vi "Teleop.vi"(10 "Match Info":T12={"Autonomous Elapsed Seconds"=0.0, "TeleOp Elapsed Seconds"=0.0, "Disabled Elapsed Seconds"=0.0, "Visited Autonomous"=FALSE, "Visited TeleOp"=FALSE, "Visited Disabled"=FALSE, "Autonomous Settings"={"Autonomous Style"=enum."Independent", "VI Refnum"=refnum}}, 11 "Call Context":T13) -> ()   [LabVIEW 2016]
doc: "This VI is called for each TeleOp packet received from the DS where the robot is not disabled. It is often used to read from the joysticks and update I/O or to update setpoints for timed control loops. It should complete and return within 20 milliseconds or it may miss DS packets."
uses:
  <vilib>/Rock Robotics/WPI/DriverStation/WPI_DriverStationDerivedRobotMode.ctl
  <vilib>/Rock Robotics/WPI/DriverStation/WPI_DriverStationMatch Info.ctl
  NavX/_TypeDefs/Flags/Z900_navX_Flags_OpStatusTypeDef.ctl
  NavX/_TypeDefs/Flags/Z900_navX_Flags_CalibrationStatusTypeDef.ctl
  NavX/_TypeDefs/Flags/Z900_navX_Flags_HardwareRevTypeDef.ctl
  NavX/_TypeDefs/Flags/Z900_navX_Flags_OmnimountConfigTypeDef.ctl
  NavX/_TypeDefs/FRIC_navX_DeviceNumbersTypeDef.ctl
  <vilib>/Rock Robotics/WPI/Utilities/WPI_GetSetVariantRefNum.vi
  <vilib>/Rock Robotics/Network Tables/NT Write Boolean Array.vi
  <vilib>/Rock Robotics/Network Tables/NT Write Numeric Array.vi
  <vilib>/Rock Robotics/Network Tables/NT Write Boolean.vi
  <vilib>/Rock Robotics/Network Tables/NT Read Boolean.vi
  <vilib>/Rock Robotics/Network Tables/NT Read Number.vi
  <vilib>/Rock Robotics/WPI/RobotDrive/WPI_RobotDriveMecanumDrive_Cartesian.vi
panel:
  out "YRPHfH 2":T1
  out "comp yaw 1":dbl format="%#.2f"
  out "Elapsed Time (s)":dbl
  out "comp yaw o":dbl format="%#.2f"
  in  "Zero Yaw":bool
  out "Displacement":T2 {"Velocity X" format="%.8f"; "Velocity Y" format="%.8f"; "Velocity Z" format="%.8f"; "Displace X" format="%.8f"; "Displace Y" format="%.8f"; "Displace Z" format="%.8f"}
  out "MPUTemp":dbl
  out "Board Information":T5 {"Board"."Hardware Revision" items=["navX-MXP"=33, "navX-Micro"=40]; "Omnimount Config" items=["DEFAULT", "X_UP", "X_DOWN", "Y_UP", "Y_DOWN", "Z_UP", "Z_DOWN"]}
  out "Linear Acceleration":cluster{"X":dbl, "Y":dbl, "Z":dbl} {"X" format="%_3g"; "Y" format="%_3g"; "Z" format="%_3g"}
  out "Offsets":T6 {"Yaw" format="%.8f"; "Quat W" format="%.8f"; "Quat X" format="%.8f"; "Quat Y" format="%.8f"; "Quat Z" format="%.8f"}
  out "Quaternion":T7 {"Quat W" format="%.8f"; "Quat X" format="%.8f"; "Quat Y" format="%.8f"; "Quat Z" format="%.8f"}
  out "Status":T10 {"OP Status" items=["INITIALIZING", "SELFTEST_IN_PROGRESS", "ERROR", "IMU_AUTOCAL_IN_PROGRESS", "NORMAL"]; "Calibration Status" items=["IMU_CAL_STATE_MASK"=3, "IMU_CAL_STATE_INPROGRESS"=0, "IMU_CAL_STATE_ACCUMULATE"=1, "IMU_CAL_STATE_COMPLETE"=2]}
  out "YRPHfH":T1
  out "Timestamp":u32
  out "Raw Values":T11 {"Accel X" format="%.8f"; "Accel Y" format="%.8f"; "Accel Z" format="%.8f"; "Gyro X" format="%.8f"; "Gyro Y" format="%.8f"; "Gyro Z" format="%.8f"; "Mag X" format="%.8f"; "Mag Y" format="%.8f"; "Mag Z" format="%.8f"}
  out "Sample Slider 0":dbl(slide) scale=0.0..5.0
  out "Sample Boolean 1":bool
  out "Sample Boolean 0":bool
  # "NavX"
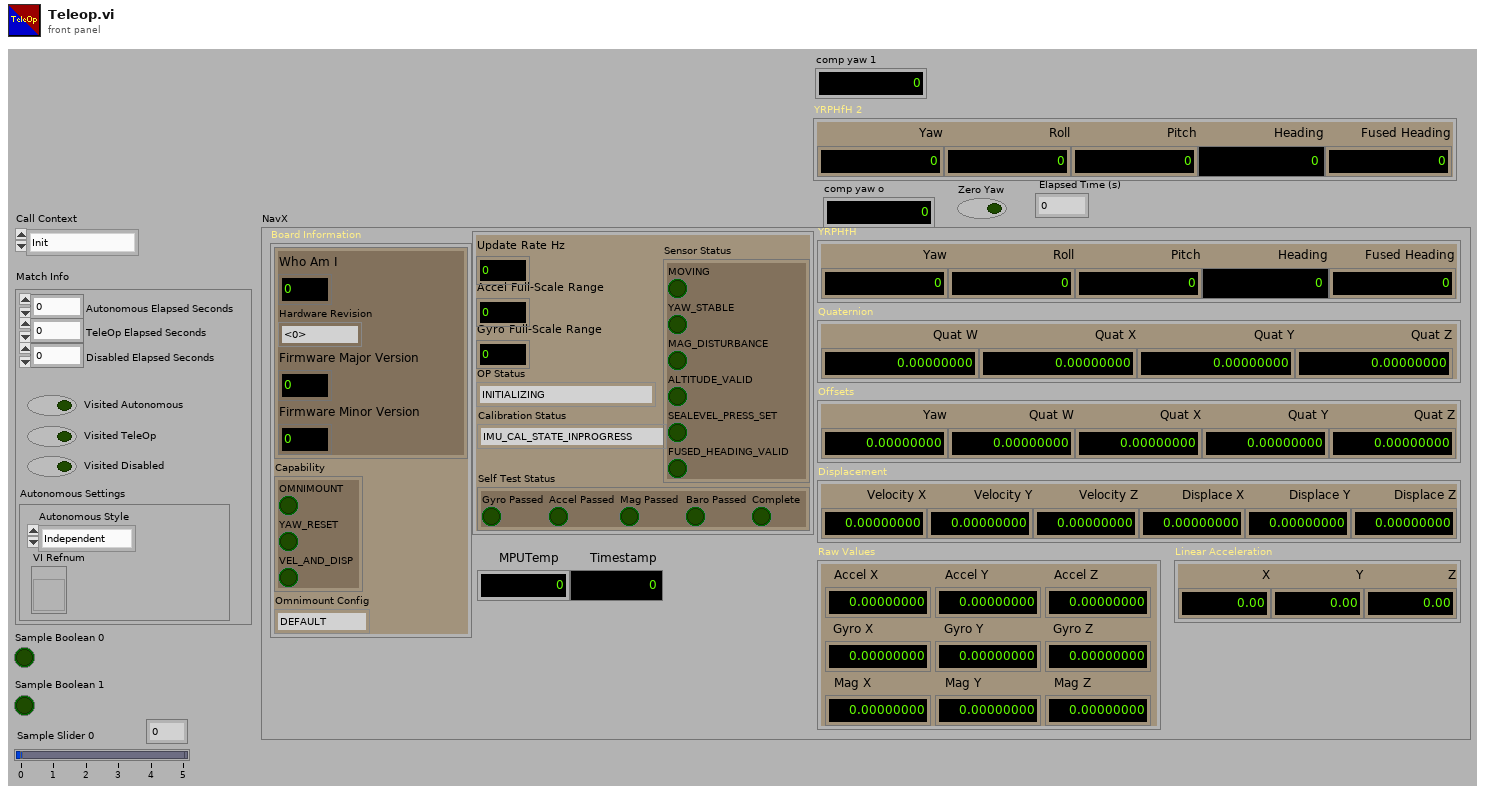
[diagram p1: front panel]
types:
  T1 = cluster{"Yaw":dbl, "Roll":dbl, "Pitch":dbl, "Heading":dbl, "Fused Heading":dbl}
  T2 = cluster{"Velocity X":dbl, "Velocity Y":dbl, "Velocity Z":dbl, "Displace X":dbl, "Displace Y":dbl, "Displace Z":dbl}
  T3 = typedef "Z900_navX_Flags_HardwareRevTypeDef.ctl" = u8
  T4 = typedef "Z900_navX_Flags_OmnimountConfigTypeDef.ctl" = u8
  T5 = cluster{"Board":cluster{"Who Am I":u8, "Hardware Revision":T3, "Firmware Major Version":u8, "Firmware Minor Version":u8}, "Capability":cluster{"OMNIMOUNT":bool, "YAW_RESET":bool, "VEL_AND_DISP":bool}, "Omnimount Config":T4}
  T6 = cluster{"Yaw":dbl, "Quat W":dbl, "Quat X":dbl, "Quat Y":dbl, "Quat Z":dbl}
  T7 = cluster{"Quat W":dbl, "Quat X":dbl, "Quat Y":dbl, "Quat Z":dbl}
  T8 = typedef "Z900_navX_Flags_OpStatusTypeDef.ctl" = u8
  T9 = typedef "Z900_navX_Flags_CalibrationStatusTypeDef.ctl" = u8
  T10 = cluster{"Update Rate Hz":u8, "Accel Full-Scale Range":u8, "Gyro Full-Scale Range":u16, "OP Status":T8, "Calibration Status":T9, "Sensor Status":cluster{"MOVING":bool, "YAW_STABLE":bool, "MAG_DISTURBANCE":bool, "ALTITUDE_VALID":bool, "SEALEVEL_PRESS_SET":bool, "FUSED_HEADING_VALID":bool}, "Self Test Status":cluster{"Gyro Passed":bool, "Accel Passed":bool, "Mag Passed":bool, "Baro Passed":bool, "Complete":bool}}
  T11 = cluster{"Accel X":dbl, "Accel Y":dbl, "Accel Z":dbl, "Gyro X":dbl, "Gyro Y":dbl, "Gyro Z":dbl, "Mag X":dbl, "Mag Y":dbl, "Mag Z":dbl}
  T12 = typedef "WPI_DriverStationMatch Info.ctl" = cluster{"Autonomous Elapsed Seconds":dbl, "TeleOp Elapsed Seconds":dbl, "Disabled Elapsed Seconds":dbl, "Visited Autonomous":bool, "Visited TeleOp":bool, "Visited Disabled":bool, "Autonomous Settings":cluster{"Autonomous Style":enum16{"Iterative", "Independent"}, "VI Refnum":refnum<vi>}}
  T13 = typedef "WPI_DriverStationDerivedRobotMode.ctl" = enum16{"Init", "Execute", "Stop"}
  T14 = typedef "FRIC_navX_DeviceNumbersTypeDef.ctl" = enum16{"Dev0", "Dev1", "Dev2", "Dev3", "Dev4", "Dev5", "Dev6", "Dev7", "Dev8", "Dev9", "Dev10"}
  T15 = typedef "WPI_JoystickDevRef.ctl" = cluster{"Device":T16}
  T16 = typedef "WPI_JoystickDeviceEnum.ctl" = enum16{"USB 0", "USB 1", "USB 2", "USB 3", "USB 4", "USB 5"}
  T17 = typedef "WPI_RobotDriveDevRef.ctl" = cluster{"DevStatus":errorcluster, "Motors[]":T18[], "Square Inputs":bool, "Max Output":dbl}
  T18 = typedef "WPI_MotorControlDeviceRef.ctl" = cluster{"DeviceStatus":errorcluster, "Type":T19, "PWM":cluster{"PWM Channel":T20, "DeadBand":T21}, "CAN":cluster{"Device Number":u8, "SetOutput VI Ref":variant, "GetOutput VI Ref":variant, "Enable VI Ref":variant, "Disable VI Ref":variant, "Data":variant}, "Invert":bool}
  T19 = typedef "WPI_MotorControlType.ctl" = enum16{"PWM", "CAN"}
  T20 = typedef "FPGA_DIOPWMChannel.ctl" = enum8{"PWM 0", "PWM 1", "PWM 2", "PWM 3", "PWM 4", "PWM 5", "PWM 6", "PWM 7", "PWM 8", "PWM 9", "PWM MXP 0", "PWM MXP 1", "PWM MXP 2", "PWM MXP 3", "PWM MXP 4", "PWM MXP 5", "PWM MXP 6", "PWM MXP 7", "PWM MXP 8", "PWM MXP 9", "Invalid"}
  T21 = typedef "WPI_PWMDeadband.ctl" = cluster{"Name":string, "maxPositivePwm":i32, "minPositivePwm":i32, "centerPwm":i32, "maxNegativePwm":i32, "minNegativePwm":i32, "angularRange":u16}
  T22 = cluster{"Velocity X":dbl, "Velocity Y":dbl, "Velocity Z":dbl, "Displacement X":dbl, "Displacement Y":dbl, "Displacement Z":dbl}
  T23 = cluster{"LinearAcceleration X":dbl, "LinearAcceleration Y":dbl, "LinearAcceleration Z":dbl}
  T24 = cluster{"Yaw Offset":dbl, "Quat Offset W":dbl, "Quat Offset X":dbl, "Quat Offset Y":dbl, "Quat Offset Z":dbl}
  T25 = cluster{"Update Rate Hz":u8, "Accelerometer Full-Scale Range":u8, "Gyro Full-Scale Range":u16, "OP Status":T8, "Calibration Status":T9, "Sensor Status":cluster{"MOVING":bool, "YAW_STABLE":bool, "MAG_DISTURBANCE":bool, "ALTITUDE_VALID":bool, "SEALEVEL_PRESS_SET":bool, "FUSED_HEADING_VALID":bool}, "Self Test Status":cluster{"Gyro Passed":bool, "Accel Passed":bool, "Mag Passed":bool, "Baro Passed":bool, "Complete":bool}}
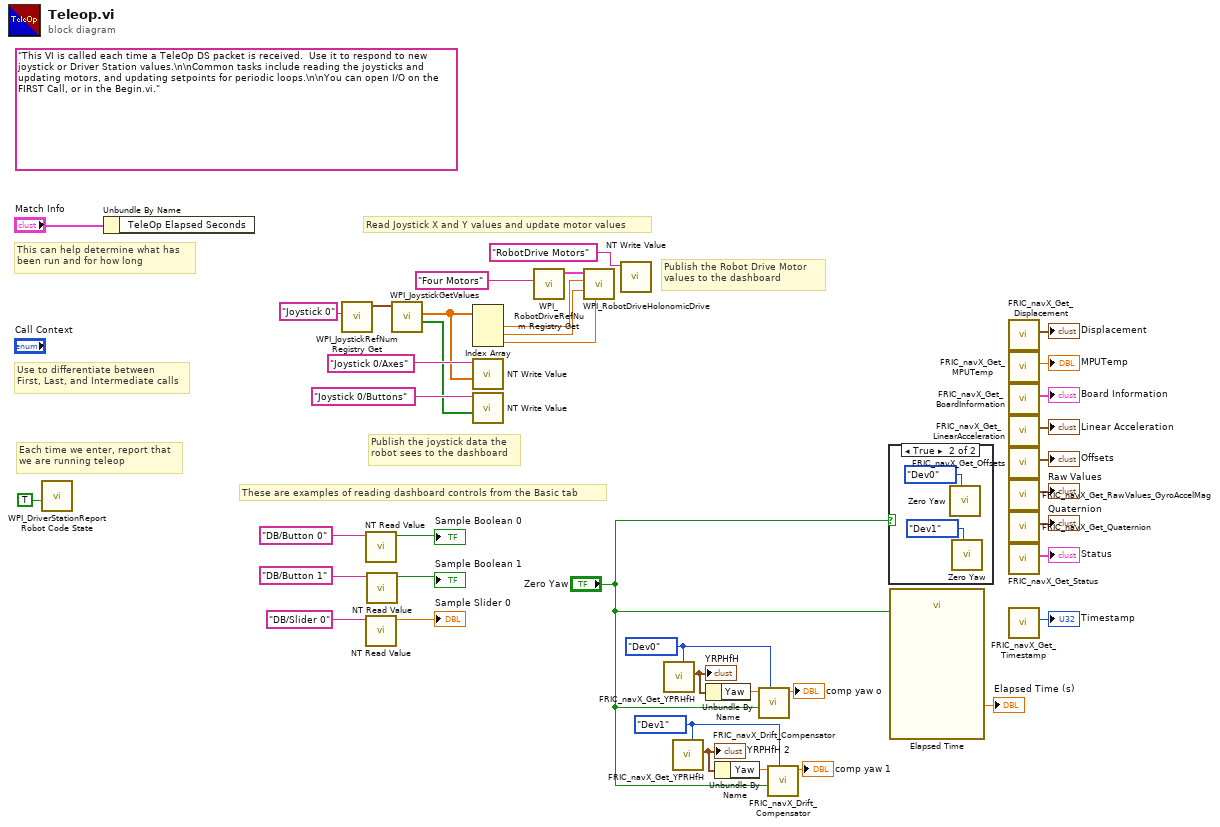
[diagram p0: block diagram]
diagram:
  w5 = FRIC_navX_DeviceNumbersTypeDef."Dev1" ("Device Number")
  w6 = FRIC_navX_DeviceNumbersTypeDef."Dev0" ("Device Number")
  (unwired) "This VI is called each time a TeleOp DS packet is received.  Use it to respond to new joystick or Driver Station values.\n\nCommon tasks include reading the joysticks and updating motors, and updating setpoints for periodic loops.\n\nYou can open I/O on the FIRST Call, or in the Begin.vi."
  # "These are examples of reading dashboard controls from the Basic tab"
  # "Publish the Robot Drive Motor\nvalues to the dashboard"
  # "Publish the joystick data the\nrobot sees to the dashboard"
  # "Each time we enter, report that\nwe are running teleop"
  # "Use to differentiate between\nFirst, Last, and Intermediate calls"
  # "This can help determine what has\nbeen run and for how long"
  # "Read Joystick X and Y values and update motor values"
  n1 = call <vilib>:"WPI_DriverStationReport Robot Code State.vi"("TeleOp"=TRUE ("Autonomous")) -> ()  [unwired: 10 in, 1 out]
  n2 = Unbundle By Name("Match Info") -> ()  [unwired: 1 out]
  n3 = call <vilib>:"WPI_JoystickRefNum Registry Get.vi"("refnum name"="Joystick 0") -> ("JoystickDevRef"=w37:T15)  [unwired: 1 in, 9 out]
  n4 = call-poly <vilib>:"NT Read Value.vi"("Name"="DB/Button 0" ("refnum name")) -> ("Boolean"=→"Sample Boolean 0":bool)  [unwired: 9 in, 1 out]
  n5 = call-poly <vilib>:"NT Read Value.vi"("Name"="DB/Slider 0" ("refnum name")) -> ("Numeric"=→"Sample Slider 0":dbl)  [unwired: 9 in, 1 out]
  n6 = call-poly <vilib>:"NT Read Value.vi"("Name"="DB/Button 1" ("refnum name")) -> ("Boolean"=→"Sample Boolean 1":bool)  [unwired: 9 in, 1 out]
  n7 = call <vilib>:"WPI_JoystickGetValues.vi"("JoystickDevRef"=w37) -> ("Buttons"=w32:bool[], "Axes"=w33:dbl[])  [unwired: 6 in, 3 out]
  n8 = Index Array(array=w33) -> (element #1=w22:dbl, element #2=w21:dbl, element #3=w20:dbl)  [unwired: 3 in]
  n9 = call-poly <vilib>:"NT Write Value.vi"("Numeric Array"=w33, "Name"="Joystick 0/Axes") -> ()  [unwired: 9 in, 1 out]
  n10 = call-poly <vilib>:"NT Write Value.vi"("Boolean Array"=w32, "Name"="Joystick 0/Buttons") -> ()  [unwired: 9 in, 1 out]
  n11 = call <vilib>:"WPI_RobotDriveRefNum Registry Get.vi"("refnum name"="Four Motors") -> ("RobotDriveDevRef"=w23:T17)  [unwired: 1 in, 9 out]
  n12 = call-poly <vilib>:"WPI_RobotDriveHolonomicDrive.vi"("Rotation"=w20, "Y"=w21, "X"=w22, "RobotDriveDevRef"=w23) -> ()  [unwired: 5 in, 3 out]
  n13 = call-poly <vilib>:"NT Write Value.vi"("Name"="RobotDrive Motors") -> ()  [unwired: 10 in, 1 out]
  n14 = call "FRIC_navX_Get_YPRHfH.vi"("Device Number"=w6) -> ("YRPHfH"=w8:T1)  [unwired: 10 in]
  "YRPHfH" <- w8
  n15 = call "FRIC_navX_Get_YPRHfH.vi"("Device Number"=w5) -> ("YRPHfH"=w3:T1)  [unwired: 10 in]
  "YRPHfH 2" <- w3
  n16 = Unbundle By Name(w8) -> ("Yaw"=w7:dbl)
  n17 = Unbundle By Name(w3) -> ("Yaw"=w4:dbl)
  n18 = call "FRIC_navX_Drift_Compensator.vi"("Device Number"=w6, "Zero Yaw"="Zero Yaw", "Raw Yaw"=w7) -> ("comp yaw"=→"comp yaw o":dbl)  [unwired: 8 in]
  n19 = call "FRIC_navX_Drift_Compensator.vi"("Device Number"=w5, "Zero Yaw"="Zero Yaw", "Raw Yaw"=w4) -> ("comp yaw"=→"comp yaw 1":dbl)  [unwired: 8 in]
  n20 = case shown="True" "Zero Yaw" {
    frame False {
    }
    frame True {
      n21 = call "Zero Yaw.vi"("Device Number"=FRIC_navX_DeviceNumbersTypeDef."Dev0") -> ()  [unwired: 11 in]
      n22 = call "Zero Yaw.vi"("Device Number"=FRIC_navX_DeviceNumbersTypeDef."Dev1") -> ()  [unwired: 11 in]
    }
  }
  n23 = call "Elapsed Time"("Reset"="Zero Yaw") -> ("Elapsed Time (s)"=→"Elapsed Time (s)":dbl)  [unwired: 11 in, 7 out]
  n24 = call "FRIC_navX_Get_Displacement.vi"() -> ("Displacement"=→"Displacement":T22)  [unwired: 11 in]
  n25 = call "FRIC_navX_Get_MPUTemp.vi"() -> ("MPUTemp"=→"MPUTemp":dbl)  [unwired: 11 in]
  n26 = call "FRIC_navX_Get_BoardInformation.vi"() -> ("Board Information"=→"Board Information":T5)  [unwired: 11 in]
  n27 = call "FRIC_navX_Get_LinearAcceleration.vi"() -> ("Linear Acceleration"=→"Linear Acceleration":T23)  [unwired: 11 in]
  n28 = call "FRIC_navX_Get_Offsets.vi"() -> ("Offsets"=→"Offsets":T24)  [unwired: 11 in]
  n29 = call "FRIC_navX_Get_RawValues_GyroAccelMag.vi"() -> ("Raw Values (out)"=→"Raw Values":T11)  [unwired: 11 in]
  n30 = call "FRIC_navX_Get_Quaternion.vi"() -> ("Quaternion"=→"Quaternion":T7)  [unwired: 11 in]
  n31 = call "FRIC_navX_Get_Status.vi"() -> ("Status"=→"Status":T25)  [unwired: 11 in]
  n32 = call "FRIC_navX_Get_Timestamp.vi"() -> ("Timestamp"=→"Timestamp":u32)  [unwired: 11 in]
